vi "Read-Panes.vi"(8 "error in (no error)":errorcluster, 11 "Panes in":refnum<class "Panes.lvclass">) -> (0 "error out":errorcluster, 2 "Panes":T1[](array[typedef]), 3 "Panes out":refnum<class "Panes.lvclass">)   [LabVIEW 2013, in "PaneToggle.lvlib" / "Panes.lvclass"]
uses:
  Panes.lvclass
  Pane-settings.ctl
  Pane-names.ctl
  Splitter-settings.ctl
  Splitter-names.ctl
  Panes.lvclass/Panes.ctl
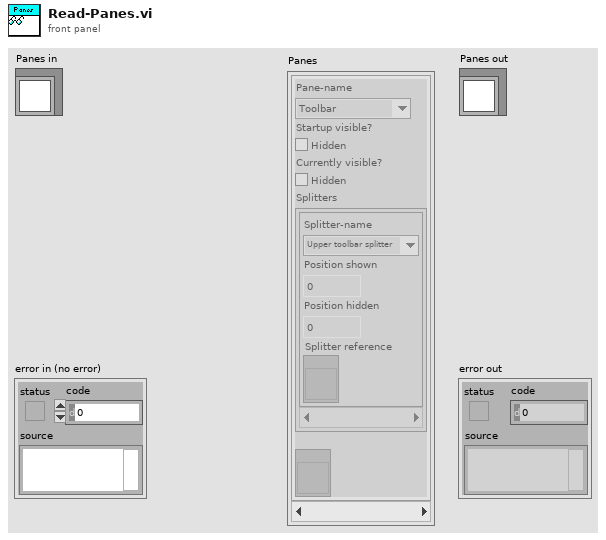
[diagram p1: front panel]
types:
  T1 = typedef "PaneToggle.lvlib/Panes.lvclass/Pane-settings.ctl" = cluster{"Pane-name":T2, "Startup visible?":bool, "Currently visible?":bool, "Splitters":T3[], "Pane-reference":refnum<vi>}
  T2 = typedef "PaneToggle.lvlib/Panes.lvclass/Pane-names.ctl" = enum16{"Toolbar", "Help bar", "Toolbar lower border", "Main panel", "Status bar upper border", "General state bar", "Information bar"}
  T3 = typedef "PaneToggle.lvlib/Panes.lvclass/Splitter-settings.ctl" = cluster{"Splitter-name":T4, "Position shown":i32, "Position hidden":i32, "Splitter reference":refnum<vi>}
  T4 = typedef "PaneToggle.lvlib/Panes.lvclass/Splitter-names.ctl" = enum16{"Upper toolbar splitter", "Help bar splitter", "Lower toolbar splitter", "Upper status bar splitter", "Lower status bar splitter", "Left status bar splitter"}
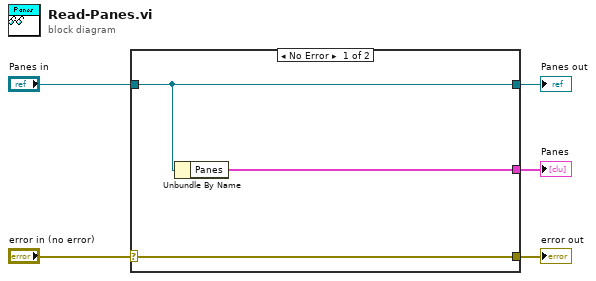
[diagram p0: block diagram]
diagram:
  n1 = case shown="No Error" "error in (no error)" {
    selector: "error in (no error)" -> [w8 w9]
    tunnel: [w8 w9] -> w4
    tunnel: [w7 w10] -> w2
    tunnel: "Panes in" -> [w7 w10]
    tunnel: [w6 _] -> w1
    frame No Error {
      n2 = Unbundle By Name(w7) -> ("Panes"=w6:T1[])
    }
    frame Error {
    }
  }
  "error out" <- w4
  "Panes out" <- w2
  "Panes" <- w1
